vi "amc_UDP Port.vi"(8 "error in (no error)":errorcluster, 11 "UDP Port Functions":T1=enum."Get") -> (0 "error out":errorcluster, 2 "UDP Port":u16=54321, 3 "UDP Port Ref":refnum<k16>)   [LabVIEW 2017]
uses:
  TypeDefs/amc_UDP Port Functions.ctl
  amc_Globals.vi
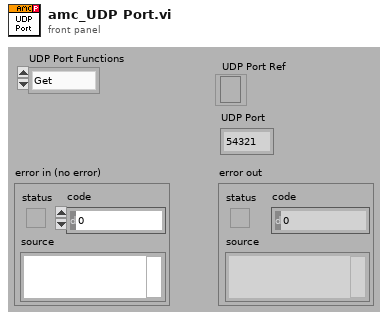
[diagram p1: front panel]
types:
  T1 = typedef "amc_UDP Port Functions.ctl" = enum16{"Init", "Get", "Close"}
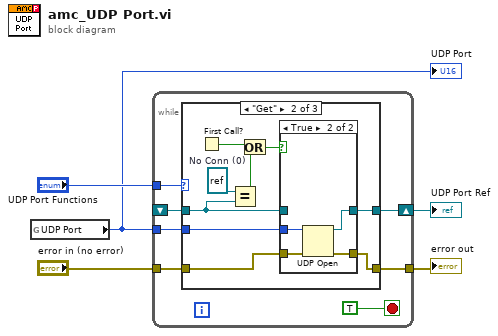
[diagram p0: block diagram]
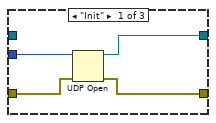
[diagram p2: hidden frame]
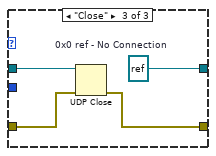
[diagram p4: hidden frame]
diagram:
  n1 = global read "amc_Globals.vi" "UDP Port"() -> (w1:u16)
  "UDP Port" <- w1
  n2 = while {
    tunnel: w1 -> [w12]
    tunnel: "UDP Port Functions" -> [w11]
    shift-right: [w9] -> w2
    shift-left: _ -> [w8]
    tunnel: [w7] -> w4
    tunnel: "error in (no error)" -> [w6]
    stop <- TRUE stop-if-true
    n3 = case shown="\"Get\"" w11 {
      tunnel: w12 -> [w16 w24 _]
      tunnel: [w15 w23 w32] -> w9
      tunnel: w8 -> [_ w22 w35]
      tunnel: [w13 w20 w34] -> w7
      tunnel: w6 -> [w14 w21 w33]
      frame "Init" {
        n4 = UDP Open(8:w14, 11:w16) -> (port=w15:refnum<k16>, 0:w13:errorcluster)  [unwired: 4 out]
      }
      frame "Get" {
        w25 = refnum<k16> refnum  # No Conn (0)
        n5 = First Call?() -> (First Call?: T/F=w19:bool)
        n6 = Equal?(x=w25, y=w22) -> (x = y?=w18:bool)
        n7 = Or(x=w19, y=w18) -> (x .or. y?=w17:bool)
        n8 = case shown="True" w17 {
          tunnel: w24 -> [_ w31]
          tunnel: [w27 w30] -> w23
          tunnel: w22 -> [w27 _]
          tunnel: w21 -> [w26 w29]
          tunnel: [w26 w28] -> w20
          frame False {
          }
          frame True {
            n9 = UDP Open(8:w29, 11:w31) -> (port=w30:refnum<k16>, 0:w28:errorcluster)  [unwired: 4 out]
          }
        }
      }
      frame "Close" {
        w32 = refnum<k16> refnum  # 0x0 ref - No Connection
        n10 = UDP Close(connection ID=w35, 8:w33) -> (error out=w34:errorcluster)  [unwired: 1 out]
      }
    }
  }
  "UDP Port Ref" <- w2
  "error out" <- w4
